vi "passTestOrganized.vi"(0 "IA State":T2, 1 "IA state":T2, 5 "IA state":T2, 7 "IA state":T2, 9 "IA state":T2, 11 "IA state":T2, 13 "IA state":T2) -> (4 "Pass state":T1)   [LabVIEW 2017]
uses:
  <extravilib>/ChannelInstances/Lossy Stream-t'AI Input.ctl'/)Channel.ctl
  Core/AI Input.ctl
  Core/AI Robot.ctl
  Intel/Functions Enum.ctl
  Intel/AttackerStates.ctl
  Core/AI Ball.ctl
  Core/Field Size.ctl
  Core/AI Judge.ctl
  Intel/Command Enum.ctl
  Util/Events/Events.ctl
  passTestStates.ctl
  <extravilib>/ChannelInstances/Lossy Stream-t'passTestStates.ctl'/Instantiate.vi
  <extravilib>/ChannelInstances/Lossy Stream-dbl/Instantiate.vi
  <extravilib>/ChannelInstances/Lossy Stream-t'AI Input.ctl'.lvlib
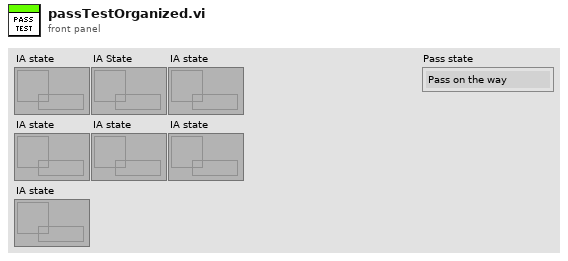
[diagram p1: front panel]
types:
  T1 = typedef "passTestStates.ctl" = enum16{"Pass on the way", "Ball stops", "Pass intercepted", "Ball out of the field", "Ball missed robot", "Need more force to pass", "Too much force", "Correct pass", "Keep ball possesion", "Robot kicked the ball", "Waiting Kick", "Invalid: same robot", "Invalid: kicker ID 999", "Invalid: Receiver ID 999", "Invalid"}
  T2 = typedef "Lossy Stream-t'AI Input.ctl'.lvlib/)Channel.ctl" = refnum<queue>
  T3 = typedef "Lossy Stream-t'passTestStates.ctl'.lvlib/)Channel.ctl" = refnum<queue>
  T4 = typedef "Lossy Stream-dbl.lvlib/)Channel.ctl" = refnum<queue>
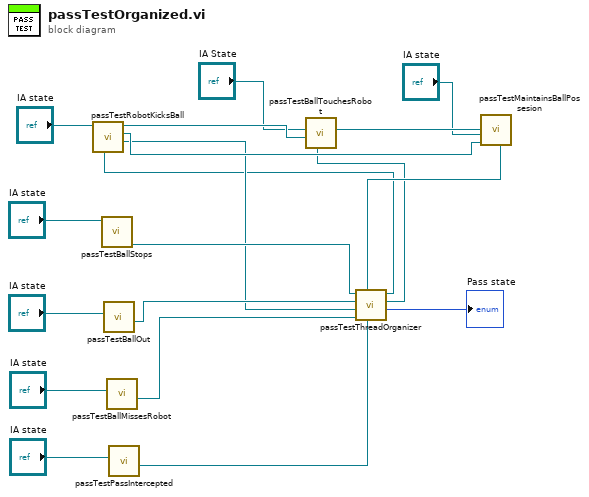
[diagram p0: block diagram]
diagram:
  n1 = call "passTestBallStops.vi"("IA state"="IA state") -> ("Result"=w9:T3)  [unwired: 10 in]
  n2 = call "passTestBallOut.vi"("IA state"="IA state") -> ("Result"=w8:T3)  [unwired: 10 in]
  n3 = call "passTestBallMissesRobot.vi"("IA state"="IA state") -> ("Result"=w6:T3)  [unwired: 10 in]
  n4 = call "passTestPassIntercepted.vi"("IA state"="IA state") -> ("Result"=w5:T3)  [unwired: 10 in]
  n5 = call "passTestRobotKicksBall.vi"("Thread organizer"=w3, "IA state"="IA state") -> ("Result"=w7:T3, 2:"Kicker robot"=w14:T4, 3:"Kicker robot"=w18:T4)  [unwired: 7 in]
  n6 = call "passTestBallTouchesRobot.vi"("Thread organizer"=w2, "Kicker robot"=w18, "IA State"="IA State") -> ("Receveing Robot"=w16:T4)  [unwired: 8 in]
  n7 = call "passTestMaintainsBallPossesion.vi"("Kicker robot"=w14, "IA state"="IA state", "Receveing robot"=w16) -> ("Result"=w4:T3)  [unwired: 8 in]
  n8 = call "passTestThreadOrganizer.vi"("Pass intercepted"=w5, "Maintains ball possesion?"=w4, "Ball missed robot"=w6, "Robot kicks ball"=w7, "Ball out"=w8, "Ball stops"=w9) -> ("Pass state"=→"Pass state":T1, 2:"Result"=w2:T3, 3:"Result"=w3:T3)  [unwired: 3 in]
